vi "Channel Handles Hierarchy to Channels Array.vi"(8 "error in":errorcluster, 11 "1553 channel handles":T2[](array[typedef]) {"messages"."timestamps" format="%.0x"; "messages"."parameters"."RxBC channel handle" format="%.0x"; "messages"."parameters"."RxRT channel handle" format="%.0x"; "messages"."parameters"."Tx channel handle" format="%.0x"}) -> (0 "error out":errorcluster, 2 "Tx Channels":T1[](array[typedef]) format="%.0x", 3 "Rx Channels":T1[](array[typedef]) format="%.0x")   [LabVIEW 2020, in "Ballard MIL-STD-1553 Engine.lvlib" / "Implementation.lvlib" / "Execution Unit.lvclass"]
uses:
  Execution Unit.lvclass
  <vilib>/NI VeriStand/Custom Device API/Custom Device Item Ref.ctl
  <vilib>/NI VeriStand/Custom Device API/Custom Device API.lvlib
  1553 Channel Handles.ctl
  Parameter Handles.ctl
  Message Handles.ctl
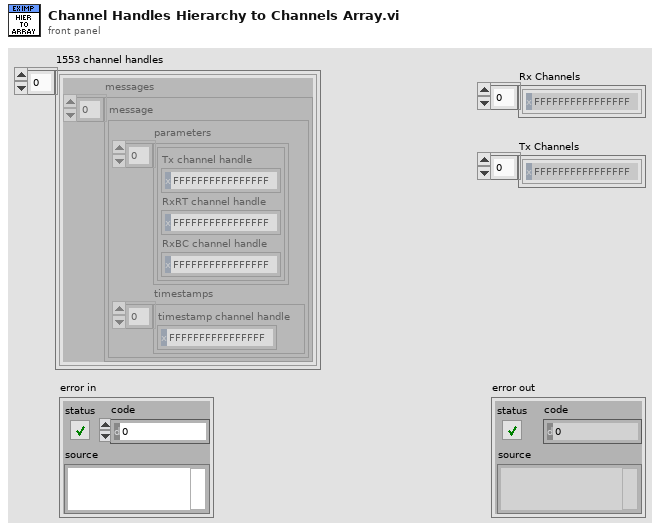
[diagram p1: front panel]
types:
  T1 = typedef "Custom Device API.lvlib/Custom Device Item Ref.ctl" = u64
  T2 = typedef "Ballard MIL-STD-1553 Engine.lvlib/Implementation.lvlib/Execution Unit.lvclass/1553 Channel Handles.ctl" = cluster{"messages":T3[]}
  T3 = typedef "Ballard MIL-STD-1553 Engine.lvlib/Implementation.lvlib/Execution Unit.lvclass/Message Handles.ctl" = cluster{"parameters":T4[], "timestamps":T1[]}
  T4 = typedef "Ballard MIL-STD-1553 Engine.lvlib/Implementation.lvlib/Execution Unit.lvclass/Parameter Handles.ctl" = cluster{"Tx channel handle":T1, "RxRT channel handle":T1, "RxBC channel handle":T1}
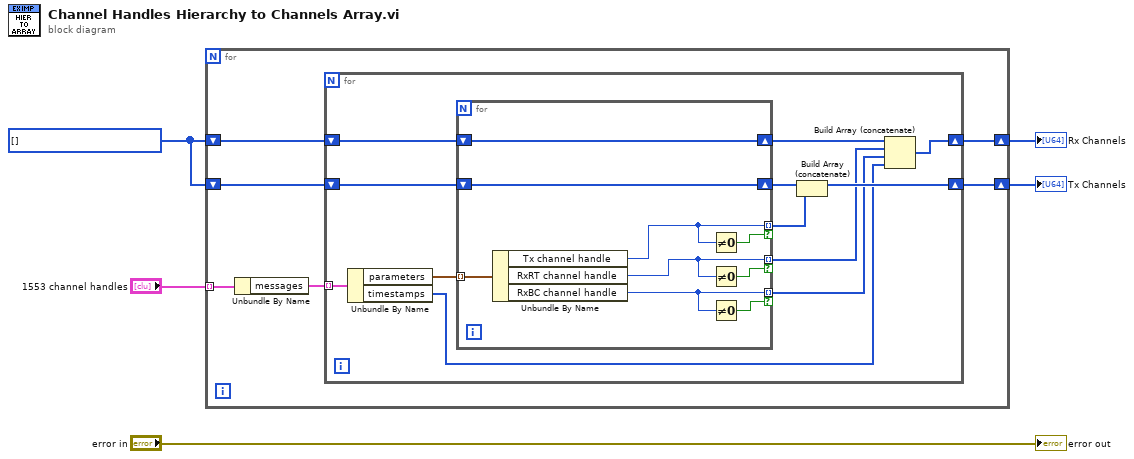
[diagram p0: block diagram]
diagram:
  w2 = T1[] [] ("Incoming Channels")
  n1 = for {
    tunnel: "1553 channel handles" -> [w11] mode=indexing
    shift-right: [w9] -> w5
    shift-left: w2 -> [w10]
    shift-right: [w7] -> w1
    shift-left: w2 -> [w8]
    n2 = Unbundle By Name(w11) -> ("messages"=w6:T3[])
    n3 = for {
      tunnel: w6 -> [w23] mode=indexing
      shift-right: [w18] -> w9
      shift-left: w10 -> [w22]
      shift-right: [w16] -> w7
      shift-left: w8 -> [w21]
      n4 = Unbundle By Name(w23) -> ("parameters"=w20:T4[], "timestamps"=w14:T1[])
      n5 = for {
        shift-right: [w31] -> w19
        shift-left: w22 -> [w31]
        tunnel: w20 -> [w32] mode=indexing
        shift-right: [w30] -> w17
        shift-left: w21 -> [w30]
        tunnel: [w26] -> w12 mode=indexing if=w27
        tunnel: [w25] -> w13 mode=indexing if=w24
        tunnel: [w28] -> w15 mode=indexing if=w29
        n6 = Unbundle By Name(w32) -> ("Tx channel handle"=w28:T1, "RxRT channel handle"=w26:T1, "RxBC channel handle"=w25:T1)
        n7 = Not Equal To 0?(x=w28) -> (x != 0?=w29:bool)
        n8 = Not Equal To 0?(x=w26) -> (x != 0?=w27:bool)
        n9 = Not Equal To 0?(x=w25) -> (x != 0?=w24:bool)
      }
      n10 = Build Array (concatenate)(w17, w15) -> (w16:T1[])
      n11 = Build Array (concatenate)(w19, w12, w13, w14) -> (w18:T1[])
    }
  }
  "Rx Channels" <- w5
  "Tx Channels" <- w1
  "error out" <- "error in"
